vi "Advance past String.vi"(7 "JSON":string, 9 "Offset":i32, 11 "State in":T1=enum."String") -> (1 "Offset past match":i32, 2 "Value start out":i32, 3 "State":T1)   [LabVIEW 2013, in "JSONtext.lvlib"]
uses:
  JSONtext.lvlib
  Parsing State.ctl
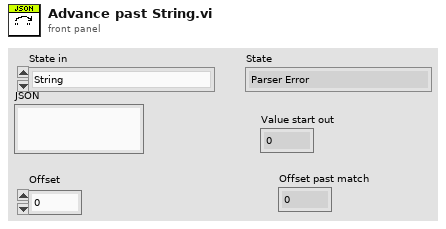
[diagram p1: front panel]
types:
  T1 = typedef "JSONtext.lvlib/Parsing State.ctl" = enum16{"Parser Error", "Object", "Array", "String", "Number/Other", "Leading Whitespace", "Object end", "Array end", "Value end"}
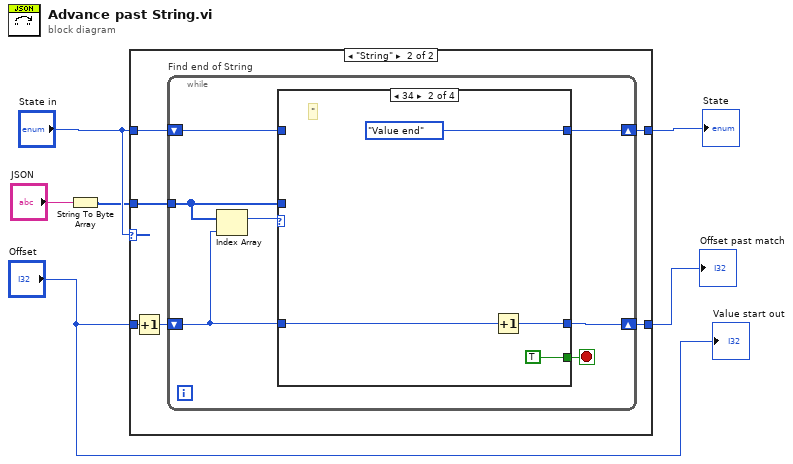
[diagram p0: block diagram]
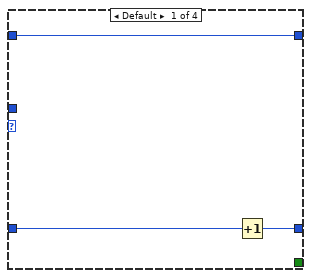
[diagram p3: hidden frame]
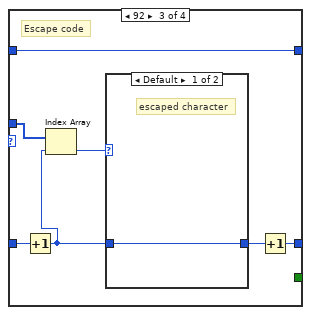
[diagram p4: hidden frame]
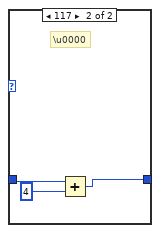
[diagram p5: hidden frame]
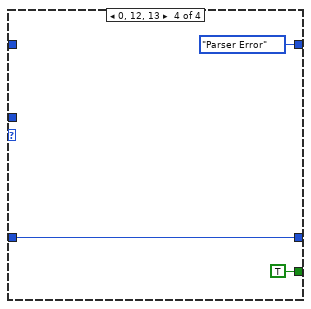
[diagram p6: hidden frame]
diagram:
  n1 = String To Byte Array(string="JSON") -> (unsigned byte array=w1:u8[])
  n2 = case shown="\"String\"" "State in" {
    tunnel: [w7 w14] -> w6
    tunnel: [w8 w13] -> w5
    tunnel: w1 -> [_ w12]
    tunnel: "State in" -> [w7 w11]
    tunnel: "Offset" -> [w8 w10]
    frame "Parser Error", Default {
    }
    frame "String" {
      n3 = Increment(x=w10) -> (x+1=w9:i32)
      n4 = while "Find end of String" {
        tunnel: w12 -> [w20]
        shift-right: [w15] -> w13
        shift-left: w9 -> [w16]
        shift-right: [w18] -> w14
        shift-left: w11 -> [w19]
        stop <- w17 stop-if-true
        n5 = Index Array(array=w20, index=w16) -> (element=w21:u8)
        n6 = case shown="34" w21 {
          tunnel: w20 -> [_ _ w33 _]
          tunnel: w19 -> [w24 _ w34 _]
          tunnel: [w24 Parsing_State."Value end" w34 Parsing_State."Parser Error"] -> w18
          tunnel: [_ TRUE _ TRUE] -> w17
          tunnel: w16 -> [w23 w26 w35 w42]
          tunnel: [w22 w25 w29 w42] -> w15
          frame Default {
            n7 = Increment(x=w23) -> (x+1=w22:i32)
          }
          frame 34 {
            # "\""
            n8 = Increment(x=w26) -> (x+1=w25:i32)
          }
          frame 92 {
            # "Escape code"
            n9 = Increment(x=w35) -> (x+1=w31:i32)
            n10 = Index Array(array=w33, index=w31) -> (element=w32:u8)
            n11 = case shown="Default" w32 {
              tunnel: w31 -> [w36 w39]
              tunnel: [w36 w37] -> w30
              frame Default {
                # "escaped character"
              }
              frame 117 {
                # "\\u0000"
                n12 = Add(x=w39, y=4) -> (x+y=w37:i32)
              }
            }
            n13 = Increment(x=w30) -> (x+1=w29:i32)
          }
          frame 0, 12, 13 {
          }
        }
      }
    }
  }
  "State" <- w6
  "Offset past match" <- w5
  "Value start out" <- "Offset"
